vi "Script Name.vi"(4 "Name":string, 6 "Name":T3, 8 "error in":errorcluster, 9 "Name Msg IO (Output).Terminal Attributes (Read)":T1, 10 "Name Msg IO (Input).Terminal Attributes (Init)":T1) -> (0 "error out":errorcluster)   [LabVIEW 2020, in "_Rescript.lvlib" / "Msg.lvlib" / "Msg.lvclass"]
uses:
  Msg.lvclass
  Name.ctl
  Terminal Attributes.ctl
  Attributes.ctl
  Find Pane.vi
  Terminal Attributes Descending Order.vi
  SubVI Terminals.vi
  <vilib>/Utility/traverseref.llb/TRef Find Object By Label.vi
  Script Control To ConPane.vi
  _Rescript.lvlib
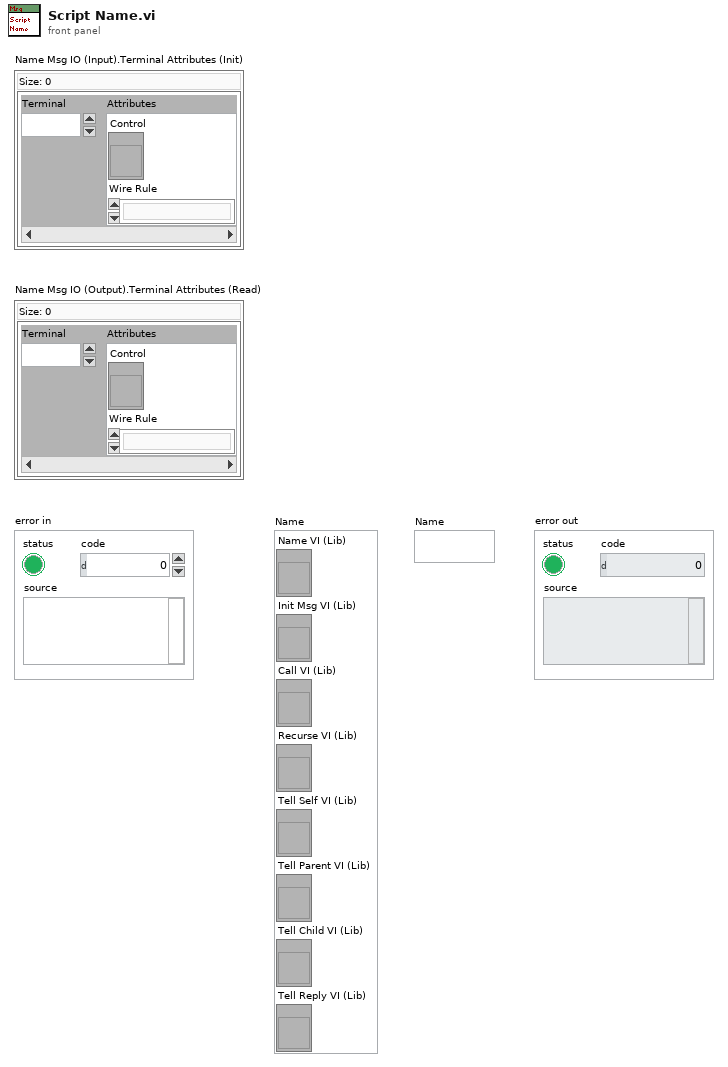
[diagram p1: front panel]
types:
  T1 = typedef "_Rescript.lvlib/Terminal Attributes.ctl" = map{i32, T2}
  T2 = typedef "_Rescript.lvlib/Attributes.ctl" = cluster{"Control":refnum<vi>, "Wire Rule":enum16{"Invalid Wire Rule", "Required", "Recommended", "Optional", "Dynamic Dispatch"}}
  T3 = typedef "_Rescript.lvlib/Msg.lvlib/Msg.lvclass/Name.ctl" = cluster{"Name VI (Lib)":refnum<vi>, "Init Msg VI (Lib)":refnum<vi>, "Call VI (Lib)":refnum<vi>, "Recurse VI (Lib)":refnum<vi>, "Tell Self VI (Lib)":refnum<vi>, "Tell Parent VI (Lib)":refnum<vi>, "Tell Child VI (Lib)":refnum<vi>, "Tell Reply VI (Lib)":refnum<vi>}
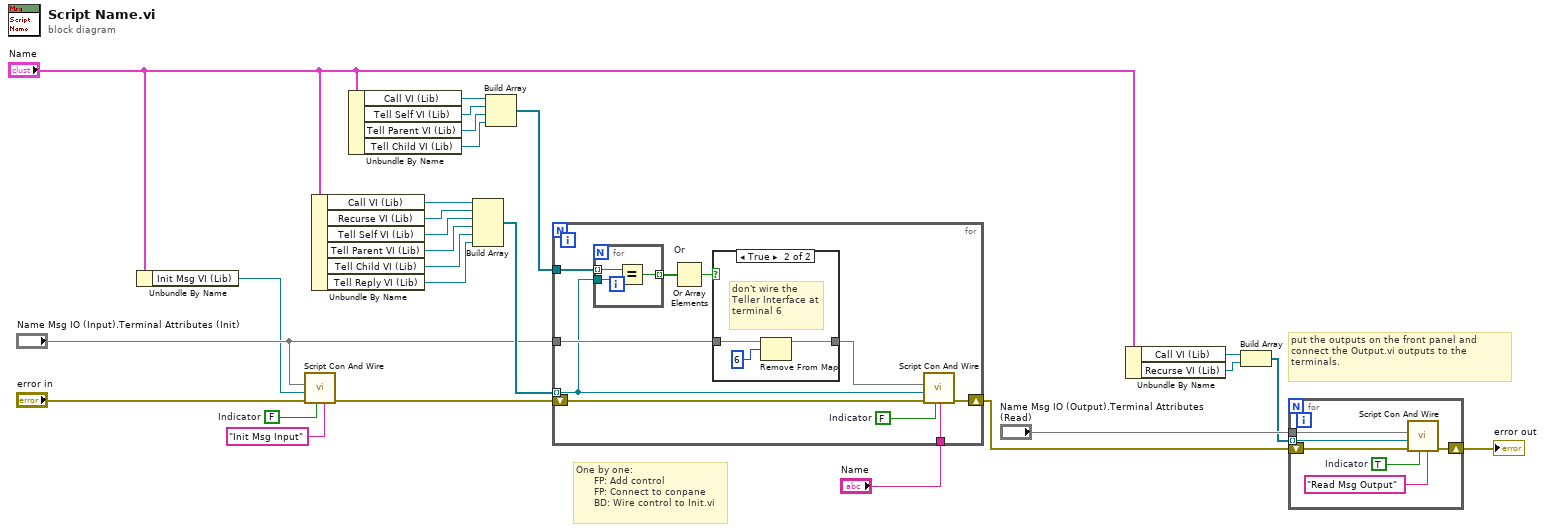
[diagram p0: block diagram]
diagram:
  w3 = FALSE  # Indicator
  # "put the outputs on the front panel and connect the Output.vi outputs to the terminals."
  # "One by one:\n      FP: Add control\n      FP: Connect to conpane\n      BD: Wire control to Init.vi"
  n1 = Unbundle By Name("Name") -> ("Init Msg VI (Lib)"=w5:refnum<vi>)
  n2 = call "Script Con And Wire.vi"("VI Name"="Init Msg Input" ("Label"), "Indicator"=w3, "error in"="error in", "VI"=w5, "Terminal Attributes"="Name Msg IO (Input).Terminal Attributes (Init)") -> ("error out"=w1:errorcluster)  [unwired: 6 in]
  n3 = Unbundle By Name("Name") -> ("Call VI (Lib)"=w16:refnum<vi>, "Recurse VI (Lib)"=w13:refnum<vi>, "Tell Self VI (Lib)"=w23:refnum<vi>, "Tell Parent VI (Lib)"=w22:refnum<vi>, "Tell Child VI (Lib)"=w21:refnum<vi>, "Tell Reply VI (Lib)"=w12:refnum<vi>)
  n4 = Unbundle By Name("Name") -> ("Call VI (Lib)"=w10:refnum<vi>, "Tell Self VI (Lib)"=w11:refnum<vi>, "Tell Parent VI (Lib)"=w8:refnum<vi>, "Tell Child VI (Lib)"=w7:refnum<vi>)
  n5 = Build Array(w16, w13, w23, w22, w21, w12) -> (w19:refnum<vi>[])
  n6 = Build Array(w10, w11, w8, w7) -> (w20:refnum<vi>[])
  n7 = for {
    shift-right: [w27] -> w26
    shift-left: w1 -> [w30]
    tunnel: w19 -> [w31] mode=indexing
    tunnel: "Name Msg IO (Input).Terminal Attributes (Init)" -> [w34]
    tunnel: w20 -> [w33]
    tunnel: "Name" -> [w28]
    w29 = FALSE  # Indicator
    n8 = for {
      tunnel: w33 -> [w42] mode=indexing
      tunnel: w31 -> [w41]
      tunnel: [w43] -> w36 mode=indexing
      n9 = Equal?(x=w42, y=w41) -> (x = y?=w43:bool)
    }
    n10 = Or Array Elements "Or"(Boolean array=w36) -> (logical OR=w35:bool)
    n11 = case shown="True" w35 {
      tunnel: w34 -> [w37 w39]
      tunnel: [w37 w38] -> w32
      frame False {
      }
      frame True {
        # "don't wire the Teller Interface at terminal 6"
        n12 = Remove From Map(10:6 ("Numeric"), 11:w39) -> (3:w38:T1)  [unwired: 2 out]
      }
    }
    n13 = call "Script Con And Wire.vi"("VI Name"=w28, "Indicator"=w29, "error in"=w30, "VI"=w31, "Terminal Attributes"=w32) -> ("error out"=w27:errorcluster)  [unwired: 6 in]
  }
  n14 = Unbundle By Name("Name") -> ("Call VI (Lib)"=w15:refnum<vi>, "Recurse VI (Lib)"=w14:refnum<vi>)
  n15 = Build Array(w15, w14) -> (w18:refnum<vi>[])
  n16 = for {
    shift-right: [w44] -> w25
    shift-left: w26 -> [w45]
    tunnel: w18 -> [w49] mode=indexing
    tunnel: "Name Msg IO (Output).Terminal Attributes (Read)" -> [w48]
    w47 = TRUE  # Indicator
    n17 = call "Script Con And Wire.vi"("VI Name"="Read Msg Output" ("Label"), "Indicator"=w47, "error in"=w45, "VI"=w49, "Terminal Attributes"=w48) -> ("error out"=w44:errorcluster)  [unwired: 6 in]
  }
  "error out" <- w25
